vi "CVT2StaticWriteTest.vi"() -> (3 "Unit Test Framework Results":T1)   [LabVIEW 2013, in "UnitTests.lvlib"]
uses:
  UnitTests.lvlib
  <vilib>/utf/common/utf_test_result_troll.ctl
  <vilib>/utf/common/utf_test_result.ctl
  <vilib>/utf/common/utf_test_result_failure.ctl
  <vilib>/utf/common/utf_test_comparison_operators.ctl
  <vilib>/utf/common/utf_vi_tag.ctl
  <vilib>/NI/Current Value Table/DataTypes/I32_Static Write.vi
  <vilib>/NI/Current Value Table/DataTypes/I32_Static Read.vi
  <vilib>/NI/Current Value Table/Type to Enum.vi
  <vilib>/NI/Current Value Table/DataTypes/I32_Type To Enum.vi
  <vilib>/NI/Current Value Table/FGVs/Tag Memory.vi
  <vilib>/NI/Current Value Table/Memory Block.vi
  <vilib>/NI/Current Value Table/DataTypes/I32_Memory Block.vi
  <vilib>/utf/NI_UnitTestFramework.lvlib
  <vilib>/NI/Current Value Table/Current Value Table.lvlib
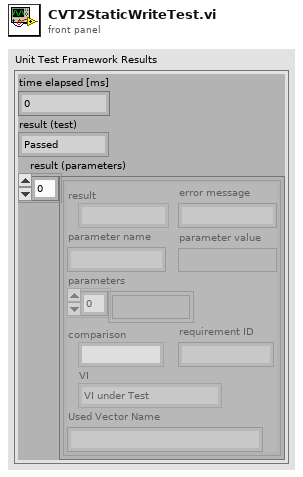
[diagram p1: front panel]
types:
  T1 = typedef "NI_UnitTestFramework.lvlib/utf_test_result_troll.ctl" = cluster{"time elapsed [ms]":u32, "result (test)":T2, "result (parameters)":T3[]}
  T2 = typedef "NI_UnitTestFramework.lvlib/utf_test_result.ctl" = enum16{"Passed", "Failed", "Error", "Skipped", "Not Processed"}
  T3 = typedef "NI_UnitTestFramework.lvlib/utf_test_result_failure.ctl" = cluster{"result":T2, "error message":string, "parameter name":string, "parameter value":variant, "parameters":variant[], "comparison":T4, "requirement ID":string, "VI":T5, "Used Vector Name":string}
  T4 = typedef "NI_UnitTestFramework.lvlib/utf_test_comparison_operators.ctl" = enum16{"=", "!=", ">", ">=", "<", "<=", "range", "symmetric tolerance", "asymmetric tolerance", "string contains", "string not contain", "array size", "string length", "array range", "by element", "array range (limit array)", "user-defined", "array contains", "array not contain", "vector length", "= (elm)", "!= (elm)", "= (case insensitive)", "!= (case insensitive)"}
  T5 = typedef "NI_UnitTestFramework.lvlib/utf_vi_tag.ctl" = enum16{"Setup VI", "VI under Test", "Teardown VI"}
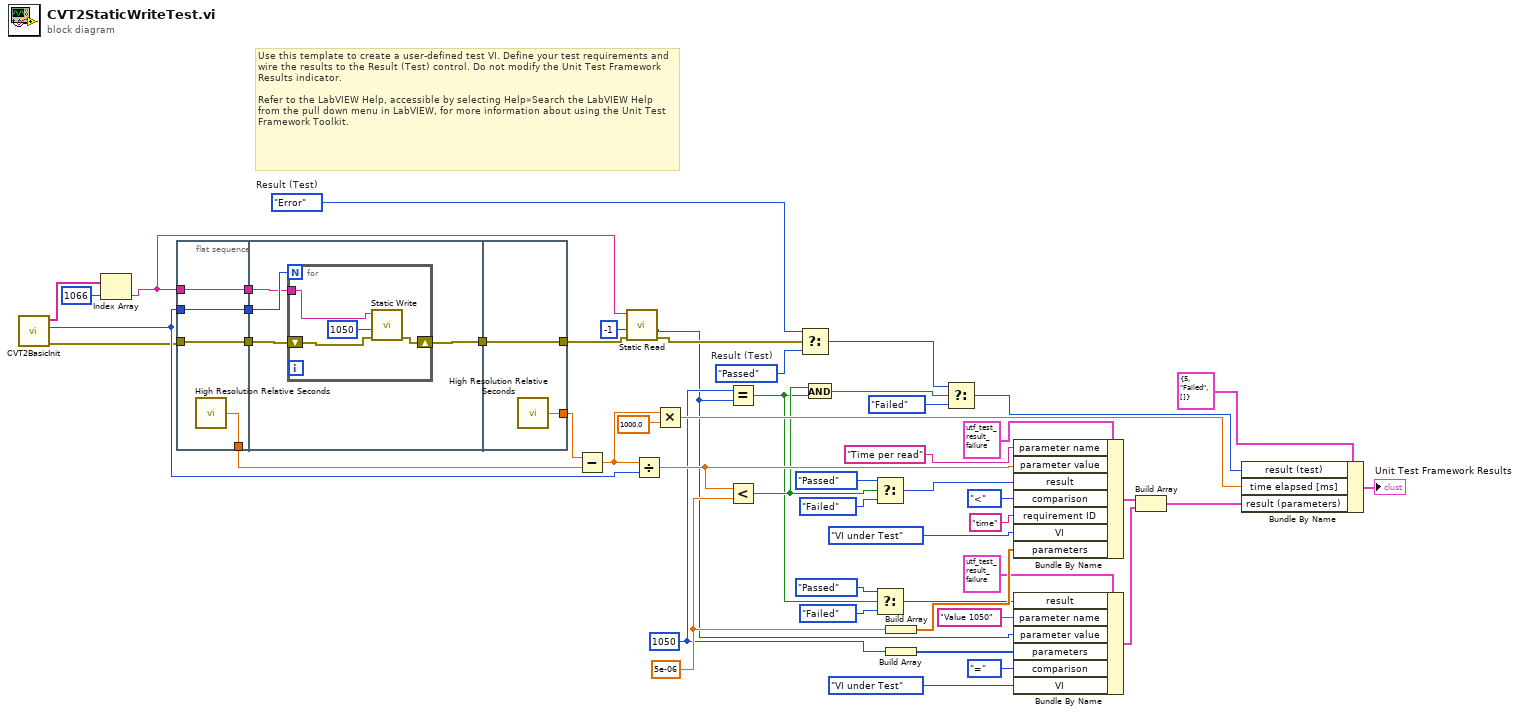
[diagram p0: block diagram]
diagram:
  w11 = 1050 ("Value")
  w25 = 5e-06 ("y")
  w46 = utf_test_result."Error"  # Result (Test)
  w45 = utf_test_result."Passed"  # Result (Test)
  # "Use this template to create a user-defined test VI. Define your test requirements and wire the results to the Result (Test) control. Do not modify the Unit Test Framework Results indicator. \n\nRefer to the LabVIEW Help, accessible by selecting Help»Search the LabVIEW Help from the pull down menu in LabVIEW, for more information about using the Unit Test Framework Toolkit."
  n1 = call "CVT2BasicInit.vi"() -> ("error out"=w9:errorcluster, "Tags per type out"=w10:i32, "names"=w8:string[])  [unwired: 9 in]
  n2 = Index Array(array=w8, index=1066) -> (element=w5:string)
  n3 = flat-sequence {
    tunnel: [w55] -> w48
    tunnel: w9 -> [w53]
    tunnel: [w54] -> w40
    tunnel: w10 -> [w54]
    tunnel: [w53] -> w39
    tunnel: w5 -> [w52]
    tunnel: [w52] -> w6
    tunnel: w40 -> [w59]
    tunnel: w39 -> [w58]
    tunnel: [w57] -> w38
    tunnel: w6 -> [w56]
    tunnel: [w65] -> w49
    tunnel: w38 -> [w64]
    tunnel: [w64] -> w3
    frame #0 {
      n4 = call <vilib>:"High Resolution Relative Seconds.vi"() -> ("relative seconds"=w55:dbl)
    }
    frame #1 {
      n5 = for {
        N: w59 -> [_]
        shift-right: [w63] -> w57
        shift-left: w58 -> [w62]
        tunnel: w56 -> [w60]
        n6 = call-poly <vilib>:"Static Write.vi"("error in (no error)"=w62, "Value"=1050, "Tag Name"=w60) -> ("error out"=w63:errorcluster)  [unwired: 8 in]
      }
    }
    frame #2 {
      n7 = call <vilib>:"High Resolution Relative Seconds.vi"() -> ("relative seconds"=w65:dbl)
    }
  }
  n8 = Subtract(x=w49, y=w48) -> (x-y=w37:dbl)
  n9 = call-poly <vilib>:"Static Read.vi"("error in (no error)"=w3, "Default"=-1, "Tag Name"=w5) -> ("error out"=w4:errorcluster, "Value"=w2:i32)  [unwired: 7 in]
  n10 = Divide(x=w37, y=w10) -> (x/y=w28:dbl)
  n11 = Multiply(x=w37, y=1000.0) -> (x*y=w41:dbl)
  n12 = Equal?(x=w11, y=w2) -> (x = y?=w13:bool)
  n13 = Less?(x=w28, y=w25) -> (x < y?=w21:bool)
  n14 = Select(t=w46, s=w4, f=w45) -> (s? t:f=w35:T2)
  n15 = And(x=w21, y=w13) -> (x .and. y?=w22:bool)
  n16 = Select(t=utf_test_result."Passed" ("result"), s=w21, f=utf_test_result."Failed" ("result")) -> (s? t:f=w29:T2)
  n17 = Select(t=utf_test_result."Passed" ("result"), s=w13, f=utf_test_result."Failed" ("result")) -> (s? t:f=w16:T2)
  n18 = Build Array(w25) -> (w24:dbl[])
  n19 = Build Array(w11) -> (w14:i32[])
  n20 = Select(t=w35, s=w22, f=utf_test_result."Failed") -> (s? t:f=w33:T2)
  n21 = Bundle By Name(cluster=T3 {"result"=enum."Passed", "error message"="", "parameter name"="", "parameter value"=variant, "parameters"=[], "comparison"=enum."=", "requirement ID"="", "VI"=enum."Setup VI", "Used Vector Name"=""} ("Unit Test Framework - result (parameters)"), "parameter name"="Time per read", "parameter value"=w28, "result"=w29, "comparison"=utf_test_comparison_operators."<", "requirement ID"="time", "VI"=utf_vi_tag."VI under Test", "parameters"=w24) -> (w44:T3)
  n22 = Bundle By Name(cluster=T3 {"result"=enum."Passed", "error message"="", "parameter name"="", "parameter value"=variant, "parameters"=[], "comparison"=enum."=", "requirement ID"="", "VI"=enum."Setup VI", "Used Vector Name"=""} ("Unit Test Framework - result (parameters)"), "result"=w16, "parameter name"="Value 1050", "parameter value"=w2, "parameters"=w14, "comparison"=utf_test_comparison_operators."=", "VI"=utf_vi_tag."VI under Test") -> (w23:T3)
  n23 = Build Array(w44, w23) -> (w43:T3[])
  n24 = Bundle By Name(cluster=T1 {"time elapsed [ms]"=5, "result (test)"=enum."Failed", "result (parameters)"=[]} ("Unit Test Framework - Result"), "result (test)"=w33, "time elapsed [ms]"=w41, "result (parameters)"=w43) -> (→"Unit Test Framework Results":T1)
